vi "Reset_Position.vi"(0 "Boolean":bool) -> ()   [LabVIEW 2013]
panel:
  in  "Position":T1(ring)
  out "P10":dbl[](array[numeric])
  out "P9":dbl[](array[numeric])
  out "P8":dbl[](array[numeric])
  out "P6":dbl[](array[numeric])
  out "P5":dbl[](array[numeric])
  out "P4":dbl[](array[numeric])
  out "P7":dbl[](array[numeric])
  out "P3":dbl[](array[numeric])
  out "P2":dbl[](array[numeric])
  out "P1":dbl[](array[numeric])
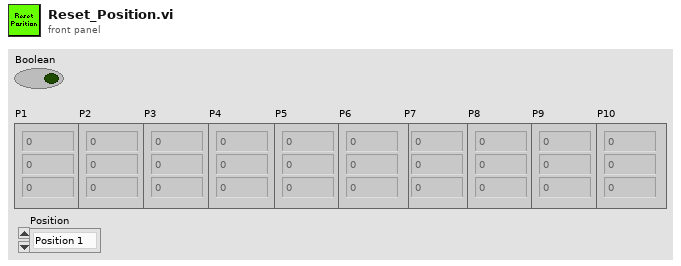
[diagram p1: front panel]
types:
  T1 = enum16{"Position 1", "Position 2", "Position 3", "Position 4", "Position 5", "Position 6", "Position 7", "Position 8", "Position 9", "Position 10"}
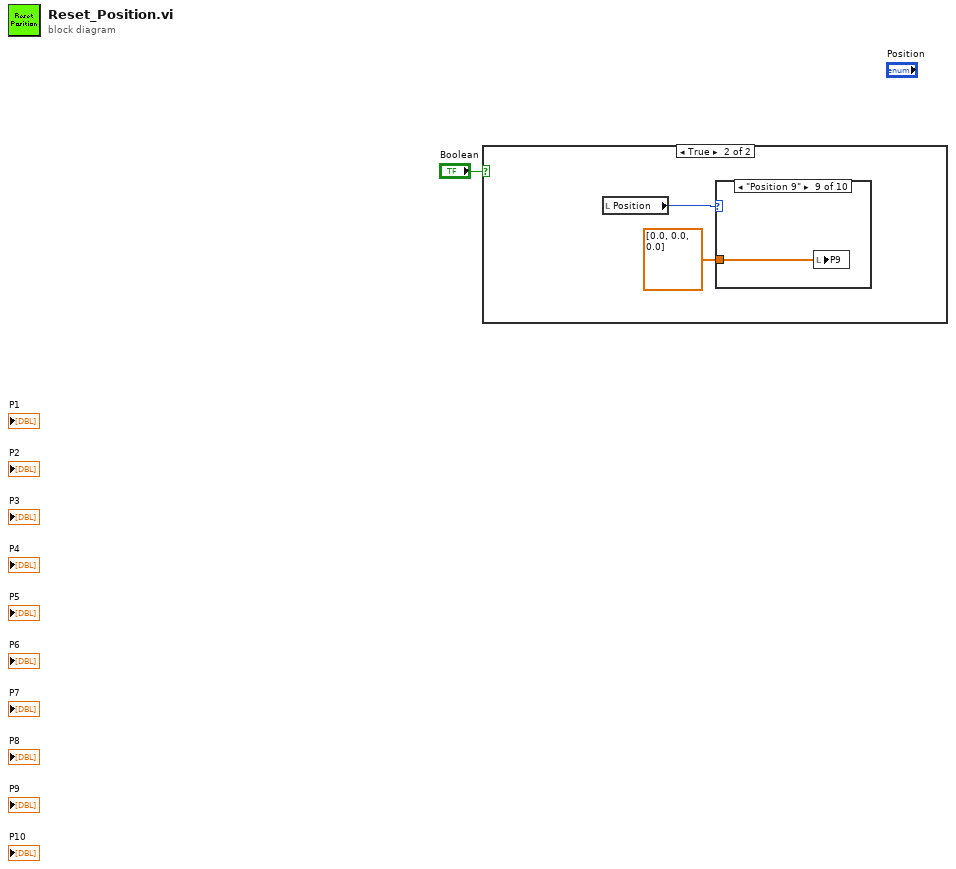
[diagram p0: block diagram]
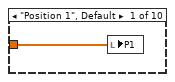
[diagram p3: hidden frame]
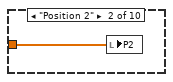
[diagram p4: hidden frame]
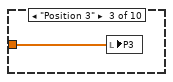
[diagram p5: hidden frame]
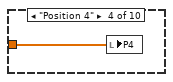
[diagram p6: hidden frame]
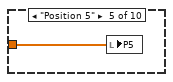
[diagram p7: hidden frame]
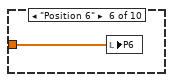
[diagram p8: hidden frame]
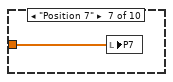
[diagram p9: hidden frame]
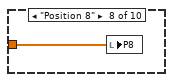
[diagram p10: hidden frame]
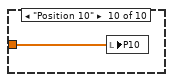
[diagram p11: hidden frame]
diagram:
  n1 = case shown="True" "Boolean" {
    frame False {
    }
    frame True {
      n2 = local read "Position"() -> (w2:T1)
      n3 = case shown="\"Position 9\"" w2 {
        tunnel: dbl[] [0.0, 0.0, 0.0] ("P1") -> [w4 w5 w6 w7 w8 w9 w10 w11 w12 w13]
        frame "Position 1", Default {
          n4 = local write "P1"(w4) -> ()
        }
        frame "Position 2" {
          n5 = local write "P2"(w5) -> ()
        }
        frame "Position 3" {
          n6 = local write "P3"(w6) -> ()
        }
        frame "Position 4" {
          n7 = local write "P4"(w7) -> ()
        }
        frame "Position 5" {
          n8 = local write "P5"(w8) -> ()
        }
        frame "Position 6" {
          n9 = local write "P6"(w9) -> ()
        }
        frame "Position 7" {
          n10 = local write "P7"(w10) -> ()
        }
        frame "Position 8" {
          n11 = local write "P8"(w11) -> ()
        }
        frame "Position 9" {
          n12 = local write "P9"(w12) -> ()
        }
        frame "Position 10" {
          n13 = local write "P10"(w13) -> ()
        }
      }
    }
  }
